vi "CCM-TDT-Read Connection Table.vi"(0 "Path In":path, 7 "TDT-Device Config":T2, 9 "Type":string, 11 "error in (no error)":errorcluster) -> (4 "Path Out":path, 8 "Table":T1[](array[typedef]), 15 "error out":errorcluster)   [LabVIEW 2020]
uses:
  PXI DAQ VIs/TDT VIs/Typedefs/TDT-Device Config.ctl
  PXI DAQ VIs/TDT VIs/Typedefs/TDT-Output source.ctl
  PXI DAQ VIs/TDT VIs/Typedefs/TDT-Device ID.ctl
  PXI DAQ VIs/TDT VIs/Typedefs/TDT-Input source.ctl
  Type Defs/CM-Connection.ctl
  <vilib>/Utility/config.llb/Read Key (String).vi
  <vilib>/Utility/config.llb/NI_LVConfig.lvlib
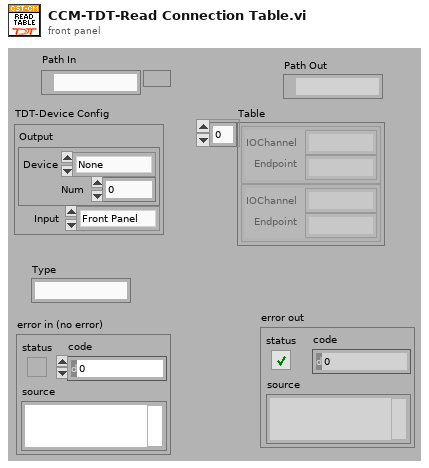
[diagram p1: front panel]
types:
  T1 = typedef "CM-Connection.ctl" = cluster{"IOChannel":string, "Endpoint":string}
  T2 = typedef "TDT-Device Config.ctl" = cluster{"Output":T3, "Input":T5}
  T3 = typedef "TDT-Output source.ctl" = cluster{"Device":T4, "Num":i32}
  T4 = typedef "TDT-Device ID.ctl" = enum16{"None", "PA5", "RP2", "RL2", "RA16", "RV8", "RX5", "RX6", "RX7", "RX8", "RZ2", "RZ5", "RZ6"}
  T5 = typedef "TDT-Input source.ctl" = enum16{"Front Panel", "RA4LI", "RA16LI"}
  T6 = typedef "NI_LVConfig.lvlib/Config Data RefNum.ctl" = refnum<k1>
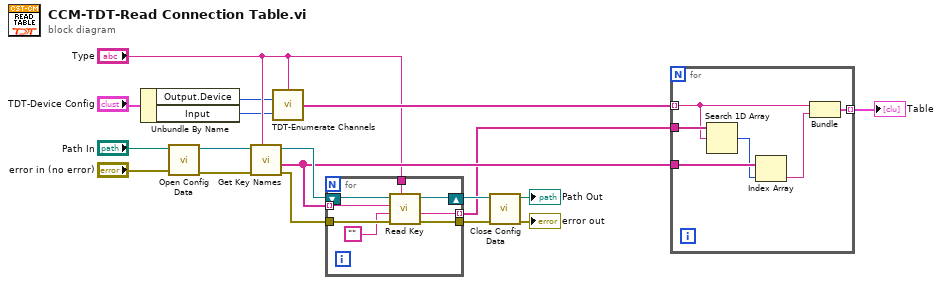
[diagram p0: block diagram]
diagram:
  n1 = Unbundle By Name("TDT-Device Config") -> ("Output.Device"=w2:T4, "Input"=w1:T5)
  n2 = call <vilib>:"Open Config Data.vi"("error in (no error)"="error in (no error)", "configuration file path"="Path In") -> ("error out"=w11:errorcluster, "refnum"=w12:T6)  [unwired: 7 in, 1 out]
  n3 = call <vilib>:"Get Key Names.vi"("section"="Type", "error in (no error)"=w11, "refnum"=w12) -> ("error out"=w9:errorcluster, "key names"=w6:string[], "refnum out"=w10:T6)  [unwired: 5 in, 1 out]
  n4 = call "TDT-Enumerate Channels.vi"("Type"="Type", "IO Device"=w2, "Input"=w1) -> ("IO Channels"=w13:string[])  [unwired: 12 in]
  n5 = for {
    tunnel: w9 -> [w24]
    tunnel: w6 -> [w25] mode=indexing
    tunnel: "Type" -> [w22]
    tunnel: [w21] -> w3 mode=indexing
    tunnel: [w19] -> w7
    shift-right: [w20] -> w8
    shift-left: w10 -> [w26]
    n6 = call-poly <vilib>:"Read Key.vi"("section"=w22, "error in (no error)"=w24, "default value"="", "key"=w25, "refnum"=w26) -> ("error out"=w19:errorcluster, "value"=w21:string, "refnum out"=w20:T6)  [unwired: 3 in, 1 out]
  }
  n7 = call <vilib>:"Close Config Data.vi"("error in (no error)"=w7, "refnum"=w8) -> ("error out"=→"error out":errorcluster, "file path"=→"Path Out":path)  [unwired: 8 in]
  n8 = for {
    tunnel: w13 -> [w29] mode=indexing
    tunnel: w3 -> [w32]
    tunnel: w6 -> [w31]
    tunnel: [w27] -> w5 mode=indexing
    n9 = Search 1D Array(1D array=w32, element=w29) -> (index of element=w30:i32)  [unwired: 1 in]
    n10 = Index Array(array=w31, index=w30) -> (element=w28:string)
    n11 = Bundle(w29, "String"=w28) -> (w27:cluster{string, "String":string})  [unwired: 1 in]
  }
  "Table" <- w5
